vi "Main.vi"() -> ()   [LabVIEW 2020]
uses:
  support/Message Queue/Message Cluster.ctl
  <vilib>/DAQmx/read.llb/DAQmx Read (Analog 1D DBL 1Chan NSamp).vi
  <extravilib>/ChannelInstances/Messenger-t'Message Queue.lvlib-Message Cluster.ctl'/Write With Abort.vi
  <extravilib>/ChannelInstances/Messenger-t'Message Queue.lvlib-Message Cluster.ctl'/Instantiate.vi
  <extravilib>/ChannelInstances/Messenger-t'Message Queue.lvlib-Message Cluster.ctl'/Endpoint.vi
  <vilib>/DAQmx/create/channels.llb/DAQmx Create Channel (AI-Voltage-Basic).vi
  <vilib>/DAQmx/configure/timing.llb/DAQmx Timing (Sample Clock).vi
  <vilib>/DAQmx/miscellaneous.llb/DAQmx Fill In Error Info.vi
  <vilib>/Utility/error.llb/Error Cluster From Error Code.vi
  <vilib>/ErrorRing/Error Ring.xnode
  support/Message Queue/Message Queue.lvlib
  <extravilib>/ChannelInstances/Messenger-t'Message Queue.lvlib-Message Cluster.ctl'.lvlib
  <resource>/objmgr/daqmx.rc
panel:
  out "Threshold Exceeded?":bool
  out "Actual Sample Rate":dbl
  in  "Threshold":dbl=4.0
  in  "Analyze Signal":bool
  in  "Sample Rate":dbl=1000.0
  in  "Generate Signal":bool
  out "RMS Result":dbl
  out "Current Consumer State":string
  out "Waveform Graph":dbl[](graph)
  in  "Exit":bool
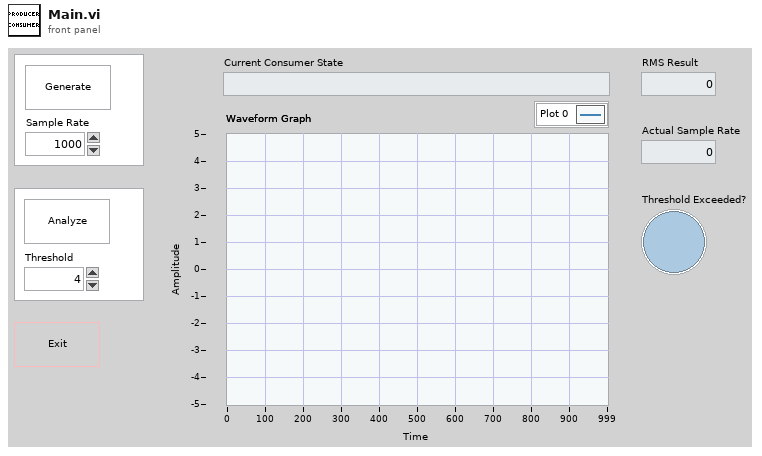
[diagram p1: front panel]
types:
  T1 = typedef "Message Queue.lvlib/Message Cluster.ctl" = cluster{"Message":string, "Message Data":variant}
  T2 = typedef "Messenger-t'Message Queue.lvlib-Message Cluster.ctl'.lvlib/))Channel.ctl" = refnum<queue>
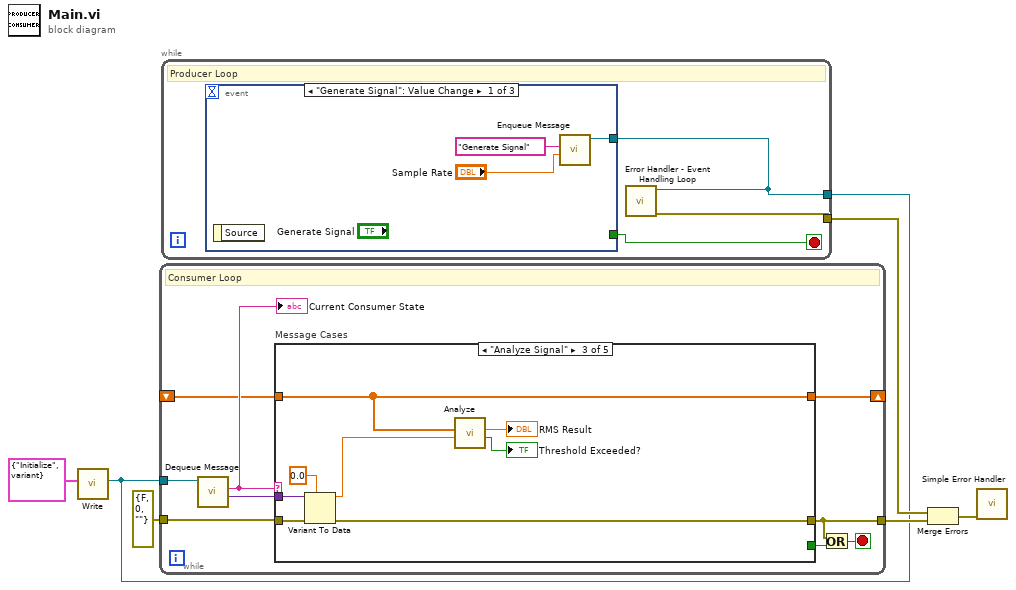
[diagram p0: block diagram]
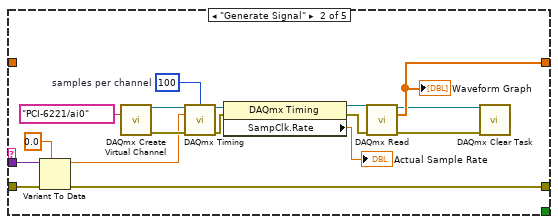
[diagram p3: hidden frame]
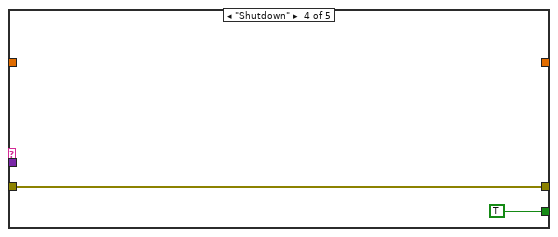
[diagram p4: hidden frame]
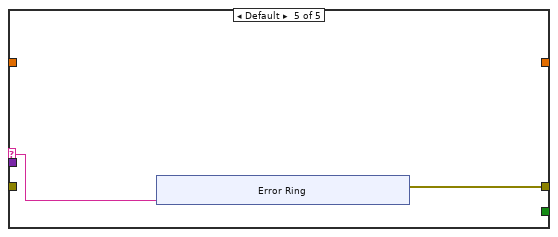
[diagram p5: hidden frame]
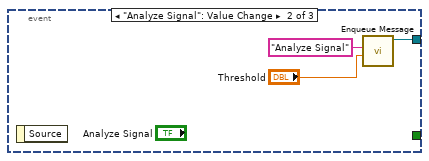
[diagram p6: hidden frame]
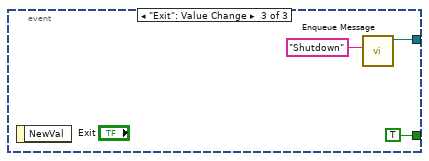
[diagram p7: hidden frame]
diagram:
  n1 = call <extravilib>:"Write.vi"("element"=T1 {"Message"="Initialize", "Message Data"=variant}) -> ("channel"=w1:T2)  [unwired: 8 in, 2 out]
  n2 = while {
    tunnel: [w11] -> w6
    tunnel: w1 -> [w14]
    tunnel: errorcluster {"status"=FALSE, "code"=0, "source"=""} ("error IO") -> [w15]
    shift-right: [w9] -> _
    shift-left: _ -> [w8]
    stop <- w13 stop-if-true
    # "Consumer Loop"
    n3 = call "Dequeue Message.vi"("channel"=w14) -> ("message data"=w7:variant, "message"=w10:string)  [unwired: 8 in, 1 out]
    "Current Consumer State" <- w10
    n4 = case "Message Cases" shown="\"Analyze Signal\"" w10 {
      selector: w10 -> [_ _ _ _ w44]
      tunnel: w15 -> [w16 w25 w37 w42 _]
      tunnel: [w16 w22 w34 w42 w45] -> w11
      tunnel: [_ _ _ TRUE ("exit confirmed") _] -> w12
      tunnel: [_ w33 w41 _ _] -> w9
      tunnel: w8 -> [_ _ w41 _ _]
      tunnel: w7 -> [_ w24 w36 _ _]
      frame "Initialize" {
        # "Initialize - All initialization work should take place in this message, since other loops can potentially enqueue messages that execute immediately after this one."
      }
      frame "Generate Signal" {
        w28 = 100  # samples per channel
        # "Something - Replace this message with functionality for your own application."
        n5 = Variant To Data(error in=w25, type=0.0, Variant=w24) -> (data=w23:dbl, error out=w22:errorcluster)
        n6 = call-poly <vilib>:"DAQmx Create Virtual Channel.vi"("physical channels"=tag "PCI-6221/ai0") -> ("task out"=w32:refnum<k21>, "error out"=w31:errorcluster)  [unwired: 13 in]
        n7 = call-poly <vilib>:"DAQmx Timing.vi"("task/channels in"=w32, "samples per channel"=w28, "rate"=w23, "error in"=w31) -> ("task out"=w20:refnum<k21>, "error out"=w19:errorcluster)  [unwired: 10 in]
        n8 = property class="DAQmx Timing"(reference=w20, error in=w19) -> (reference out=w17:refnum<k21>, error out=w18:errorcluster, "SampClk.Rate"=→"Actual Sample Rate":dbl)
        n9 = call-poly <vilib>:"DAQmx Read.vi"("task/channels in"=w17, "error in"=w18) -> ("task out"=w30:refnum<k21>, "data"=w33:dbl[], "error out"=w29:errorcluster)  [unwired: 11 in]
        "Waveform Graph" <- w33
        n10 = call <vilib>:"DAQmx Clear Task.vi"("task in"=w30, "error in"=w29) -> ()  [unwired: 13 in, 1 out]
      }
      frame "Analyze Signal" {
        n11 = Variant To Data(error in=w37, type=0.0, Variant=w36) -> (data=w35:dbl, error out=w34:errorcluster)
        n12 = call "Analyze.vi"("Threshold (rms)"=w35, "Data (1D DBL)"=w41) -> ("Threshold Exceeded?"=→"Threshold Exceeded?":bool, "RMS Result"=→"RMS Result":dbl)  [unwired: 8 in]
      }
      frame "Shutdown" {
        # "Something Else - Replace this message with functionality for your own application."
      }
      frame Default {
        # "'Default' case only runs if there is a message that isn't defined in any of the other cases.  Output a programming error."
        n13 = xnode "Error Ring"("parameter 0"=w44) -> ("error out"=w45:errorcluster)
      }
    }
    n14 = Or(x=w11, y=w12) -> (x .or. y?=w13:bool)
  }
  n15 = while {
    tunnel: [w54] -> w3
    tunnel: w1 -> [w53]
    stop <- w55 stop-if-true
    # "Producer Loop"
    n16 = event shown="[0] \"Generate Signal\": Value Change" {
      selector: _ -> [_ _ _]
      dyn-events: _ -> [_ _ _]
      timeout: _ -> [_ _ _]
      tunnel: [_ _ TRUE ("exit confirmed")] -> w55
      tunnel: [w58 w60 w63] -> w53
      event "Generate Signal": Value Change {
        n17 = event-data() -> ()  [unwired: 1 in, 1 out]
        n18 = call "Enqueue Message.vi"("data (empty)"="Sample Rate", "message"="Generate Signal" ("Message")) -> ("channel"=w58:T2)  [unwired: 9 in]
      }
      event "Analyze Signal": Value Change {
        n19 = event-data() -> ()  [unwired: 1 in, 1 out]
        n20 = call "Enqueue Message.vi"("data (empty)"="Threshold", "message"="Analyze Signal" ("Message")) -> ("channel"=w60:T2)  [unwired: 9 in]
      }
      event "Exit": Value Change {
        n21 = event-data() -> ()  [unwired: 1 in, 1 out]
        n22 = call "Enqueue Message.vi"("message"="Shutdown" ("Message")) -> ("channel"=w63:T2)  [unwired: 10 in]
      }
    }
    n23 = call "Error Handler - Event Handling Loop.vi"("channel"=w53) -> ("dup error in"=w54:errorcluster)  [unwired: 10 in]
  }
  n24 = Merge Errors(w3, w6) -> (w2:errorcluster)
  n25 = call <vilib>:"Simple Error Handler.vi"("error in (no error)"=w2) -> ()  [unwired: 4 in, 5 out]
